vi "_DServerGetRawDeviceProperty.vi"(2 "property_name":string, 3 "device_name":string, 4 "error in":errorcluster) -> (0 "property_value":T1={"Name"="", "Data"=[], "Tango Data Type"=enum."UNKNOWN_DATA_TYPE"}, 1 "error out":errorcluster)   [LabVIEW 2014, in "tango.lvlib"]
uses:
  tango.lvlib
  Client Request Handling/Typedefs/_DeviceProperty.ctl
  Common VIs/Typedefs/_AttributeDataType_t.ctl
  tango_binding.so
panel:
  in  "device property":T1
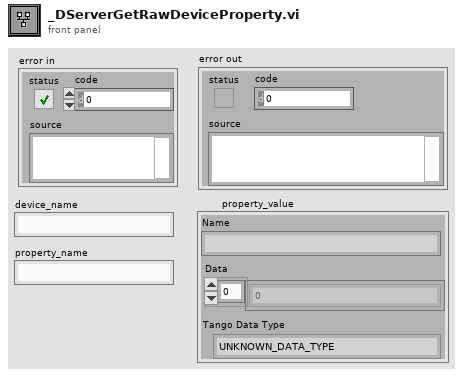
[diagram p1: front panel]
types:
  T1 = typedef "tango.lvlib/_DeviceProperty.ctl" = cluster{"Name":string, "Data":u8[], "Tango Data Type":T2}
  T2 = typedef "tango.lvlib/_AttributeDataType_t.ctl" = enum16{"STATE_SCA", "STATE_SPE", "STATE_IMG", "STRING_SCA", "STRING_SPE", "STRING_IMG", "BOOL_SCA", "BOOL_SPE", "BOOL_IMG", "UCHAR_SCA", "UCHAR_SPE", "UCHAR_IMG", "SHORT_SCA", "SHORT_SPE", "SHORT_IMG", "USHORT_SCA", "USHORT_SPE", "USHORT_IMG", "LONG_SCA", "LONG_SPE", "LONG_IMG", "ULONG_SCA", "ULONG_SPE", "ULONG_IMG", "LONG64_SCA", "LONG64_SPE", "LONG64_IMG", "ULONG64_SCA", "ULONG64_SPE", "ULONG64_IMG", "FLOAT_SCA", "FLOAT_SPE", "FLOAT_IMG", "DOUBLE_SCA", "DOUBLE_SPE", "DOUBLE_IMG", "ENUM_SCA", "UNKNOWN_DATA_TYPE"}
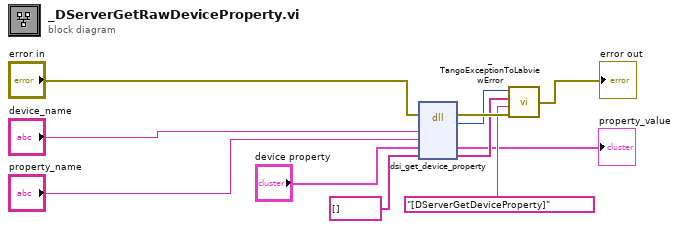
[diagram p0: block diagram]
diagram:
  n1 = dll-call lib="tango_binding.*" fn="dsi_get_device_property"(error in="error in", "device_name"="device_name", "property_name"="property_name", "property_value"="device property", "error_stack"=string[] [] ("error stack")) -> (error out=w8:errorcluster, "return type"=w6:i32, "property_value"=→"property_value":T1, "error_stack"=w7:string[])  [unwired: 4 in, 1 out]
  n2 = call "_TangoExceptionToLabviewError.vi"("error in"=w8, "location"="[DServerGetDeviceProperty]", "error stack"=w7, "error code"=w6) -> ("error out"=→"error out":errorcluster)
